vi "Read Processing buffer refs.vi"(8 "error in (no error)":errorcluster, 11 "Buffers in":refnum<class "CV-Buffers.lvclass">) -> (0 "error out":errorcluster, 2 "Processing buffer refs":T1[][](array[typedef]), 3 "Buffers out":refnum<class "CV-Buffers.lvclass">)   [LabVIEW 2013, in "CameraVision.lvlib" / "CV-Buffers.lvclass"]
uses:
  CV-Buffers.lvclass
  <vilib>/vision/Image Controls.llb/IMAQ Image.ctl
  CV-Buffers.lvclass/CV-Buffers.ctl
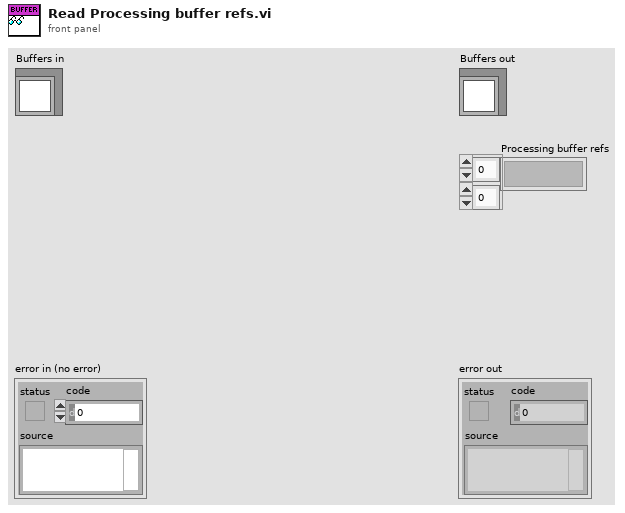
[diagram p1: front panel]
types:
  T1 = typedef "IMAQ Image.ctl" = refnum<image>
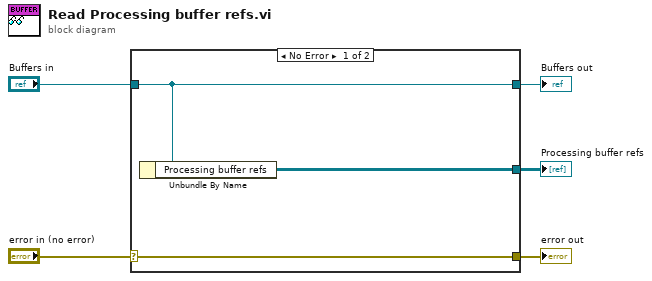
[diagram p0: block diagram]
diagram:
  n1 = case shown="No Error" "error in (no error)" {
    selector: "error in (no error)" -> [w8 w9]
    tunnel: [w8 w9] -> w4
    tunnel: [w7 w10] -> w2
    tunnel: "Buffers in" -> [w7 w10]
    tunnel: [w6 _] -> w1
    frame No Error {
      n2 = Unbundle By Name(w7) -> ("Processing buffer refs"=w6:T1[][])
    }
    frame Error {
    }
  }
  "error out" <- w4
  "Buffers out" <- w2
  "Processing buffer refs" <- w1
